vi "1.Basic demo.vi"() -> ()   [LabVIEW 2022 SP3]
uses:
  UnderAutomation.UniversalRobots/UnderAutomation.UniversalRobots.lvlib
  C:/Users/fg/Documents/UniversalRobots.vi/LabVIEW_2023/UnderAutomation.UniversalRobots/lib/UnderAutomation.UniversalRobots.dll
  LabVIEW_2023/UnderAutomation.UniversalRobots/lib/UnderAutomation.UniversalRobots.dll
panel:
  out "Configurable0":bool
  out "error out":errorcluster
  out "Waveform 1":dbl(graph)
  out "Connected":bool
  in  "stop":bool
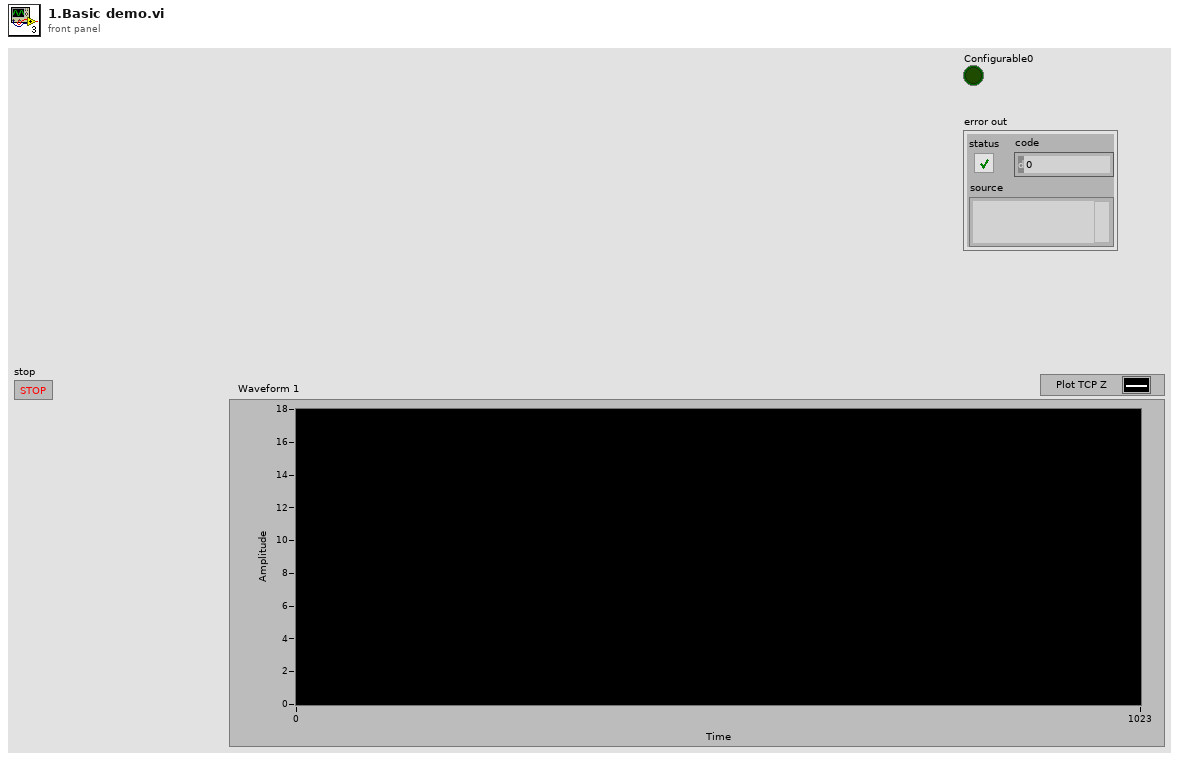
[diagram p1: front panel]
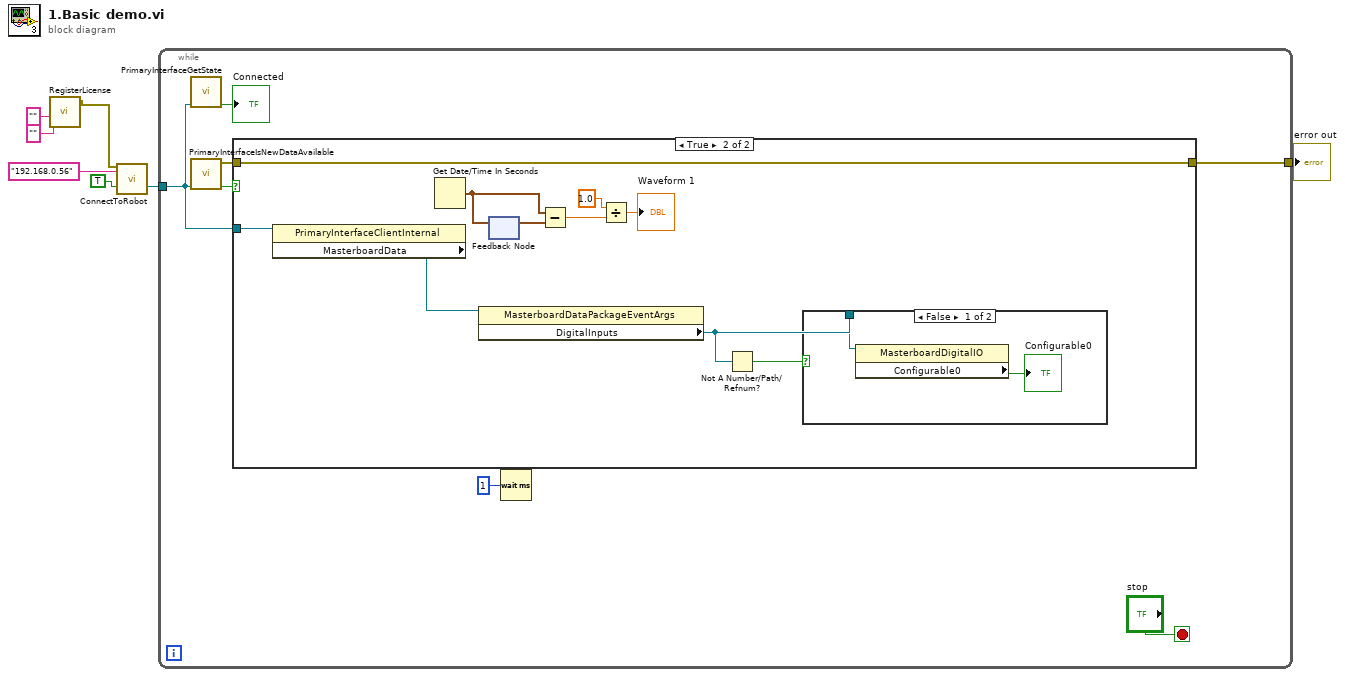
[diagram p0: block diagram]
diagram:
  n1 = call "RegisterLicense.vi"("key"="", "licensee"="") -> ("error out"=w3:errorcluster)  [unwired: 6 in, 2 out]
  n2 = call "ConnectToRobot.vi"("error in"=w3, "ip"="192.168.0.56", "Enable Primary Interface"=TRUE) -> ("PrimaryInterface"=w4:refnum<k24>)  [unwired: 11 in, 5 out]
  n3 = while {
    tunnel: w4 -> [w10]
    tunnel: [w8] -> w5
    stop <- "stop" stop-if-true
    n4 = call "PrimaryInterfaceGetState.vi"("PrimaryInterface"=w10) -> ("Connected"=→"Connected":bool)  [unwired: 9 in, 1 out]
    n5 = call "PrimaryInterfaceIsNewDataAvailable.vi"("PrimaryInterface"=w10) -> ("Data available"=w11:bool, "error out"=w9:errorcluster)  [unwired: 9 in]
    n6 = case shown="True" w11 {
      tunnel: w10 -> [_ w20]
      tunnel: w9 -> [w15 w18]
      tunnel: [w15 w18] -> w8
      frame False {
      }
      frame True {
        n7 = property class="PrimaryInterfaceClientInternal"(reference=w20) -> ("MasterboardData"=w19:refnum<k24>)  [unwired: 1 in, 2 out]
        n8 = Get Date/Time In Seconds() -> (seconds since 1Jan1904=w25:timestamp)
        n9 = property class="MasterboardDataPackageEventArgs"(reference=w19) -> ("DigitalInputs"=w16:refnum<k24>)  [unwired: 1 in, 2 out]
        n10 = feedback #1() -> (w24:timestamp)  [unwired: 1 in]
        n11 = feedback-in #1(w25) -> ()
        n12 = Subtract(x=w25, y=w24) -> (x-y=w23:dbl)
        n13 = Divide(x=1.0, y=w23) -> (x/y=→"Waveform 1":dbl)
        n14 = Not A Number/Path/Refnum?(number/path/refnum=w16) -> (NaN/Path/Refnum?=w17:bool)
        n15 = case shown="False" w17 {
          tunnel: w16 -> [w27 _]
          frame False {
            n16 = property class="MasterboardDigitalIO"(reference=w27) -> ("Configurable0"=→"Configurable0":bool)  [unwired: 1 in, 2 out]
          }
          frame True {
          }
        }
      }
    }
    n17 = Wait (ms)(milliseconds to wait=u32 1) -> ()  [unwired: 1 out]
  }
  "error out" <- w5
